vi "TCP Named Service - Server.vi"() -> ()   [LabVIEW 2015]
doc: "Creates a named service and listens on the first available port. When a client connects to the service, it sends a response string to the client."
panel:
  in  "MirrorCoverMotor":T1
  in  "Message to Send":string="You are currently accessing TCP Named Service - Server.vi from client %s on port %d."
  in  "Stop":bool
  # "Overview: Demonstrates the use of the TCP functions to initialize a named TCP service that can send data to a client VI.\nInstructions:\n1. Run the VI.\n2. Open TCP Named Service - Client.vi and follow the instructions on its front panel.\n3. Click Stop to stop the VI."
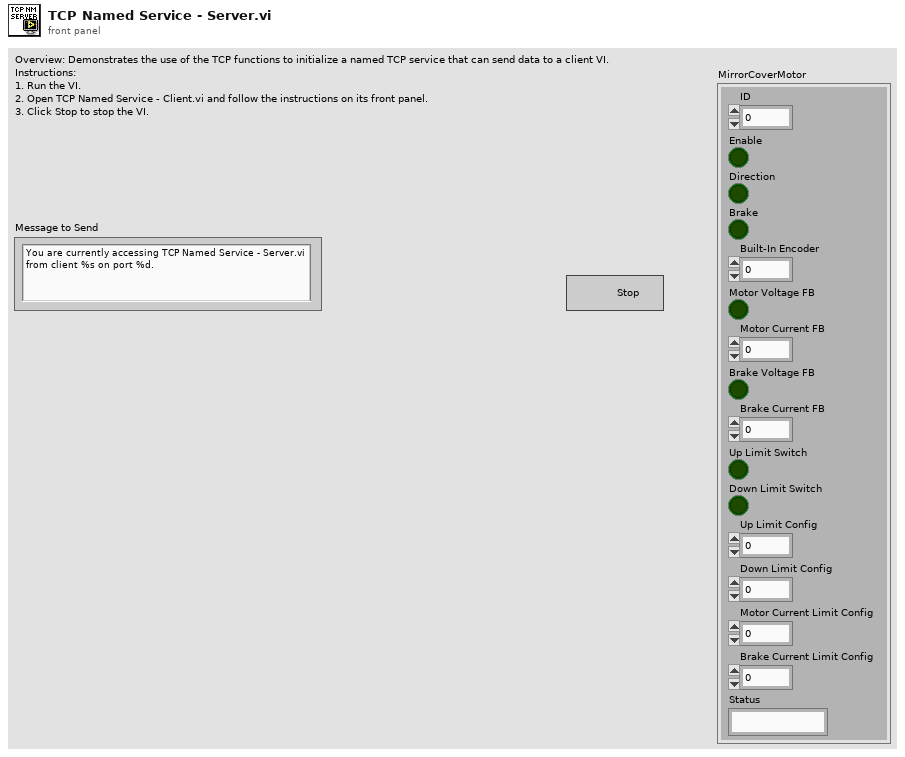
[diagram p1: front panel]
types:
  T1 = cluster{"ID":i32, "Enable":bool, "Direction":bool, "Brake":bool, "Built-In Encoder":u64, "Motor Voltage FB":bool, "Motor Current FB":u64, "Brake Voltage FB":bool, "Brake Current FB":u64, "Up Limit Switch":bool, "Down Limit Switch":bool, "Up Limit Config":u64, "Down Limit Config":u64, "Motor Current Limit Config":u64, "Brake Current Limit Config":u64, "Status":string}
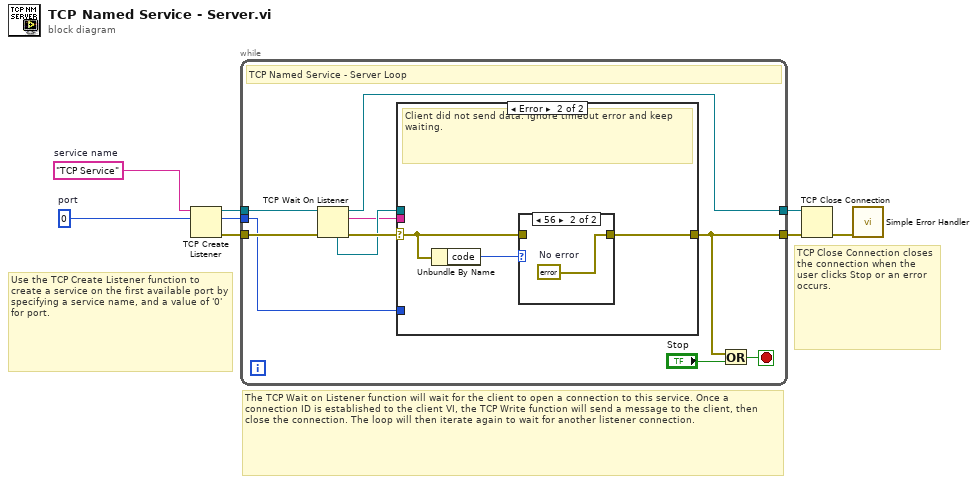
[diagram p0: block diagram]
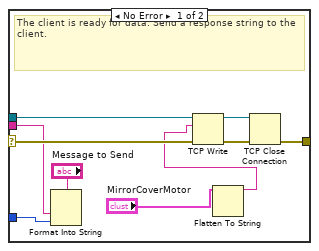
[diagram p2: hidden frame]
diagram:
  w2 = u16 0  # port
  w1 = "TCP Service"  # service name
  # "TCP Close Connection closes the connection when the user clicks Stop or an error occurs."
  # "The TCP Wait on Listener function will wait for the client to open a connection to this service. Once a connection ID is established to the client VI, the TCP Write function will send a message to the client, then close the connection. The loop will then iterate again to wait for another listener connection."
  # "Use the TCP Create Listener function to create a service on the first available port by specifying a service name, and a value of '0' for port."
  n1 = TCP Create Listener(10:w2, 11:w1) -> (0:w7:errorcluster, 2:w4:u16, 3:w8:refnum<k5>)  [unwired: 3 in]
  n2 = while {
    tunnel: [w11] -> w5
    tunnel: w8 -> [w18]
    tunnel: w7 -> [w16]
    tunnel: [w9] -> w6
    tunnel: w4 -> [w14]
    stop <- w13 stop-if-true
    # "TCP Named Service - Server Loop"
    n3 = TCP Wait On Listener(8:w16, 11:w18) -> (0:w17:errorcluster, 2:w10:string, 3:w9:refnum<k5>, 4:w15:refnum<k5>)  [unwired: 2 in, 1 out]
    n4 = case shown="Error" w17 {
      selector: w17 -> [w28 w31]
      tunnel: [w23 w29] -> w11
      tunnel: w15 -> [w26 _]
      tunnel: w14 -> [w27 _]
      tunnel: w10 -> [w25 _]
      frame No Error {
        # "The client is ready for data. Send a response string to the client."
        n5 = Format Into String(initial string="Message to Send", w25, w27) -> ()  [unwired: 2 in, 2 out]
        n6 = Flatten To String(anything="MirrorCoverMotor") -> (data string=w19:string)  [unwired: 3 in, 2 out]
        n7 = TCP Write(connection ID=w26, data in=w19, error in (no error)=w28) -> (connection ID out=w22:refnum<k5>, error out=w24:errorcluster)  [unwired: 1 in, 1 out]
        n8 = TCP Close Connection(connection ID=w22, error in (no error)=w24) -> (error out=w23:errorcluster)  [unwired: 1 in, 1 out]
      }
      frame Error {
        # "Client did not send data. Ignore timeout error and keep waiting."
        n9 = Unbundle By Name(w31) -> ("code"=w30:i32)
        n10 = case shown="56" w30 {
          tunnel: w31 -> [w32 _]
          tunnel: [w32 w33] -> w29
          frame Default {
          }
          frame 56 {
            w33 = errorcluster {"status"=FALSE, "code"=0, "source"=""}  # No error
          }
        }
      }
    }
    n11 = Or(x=w11, y="Stop") -> (x .or. y?=w13:bool)
  }
  n12 = TCP Close Connection(connection ID=w6, error in (no error)=w5) -> (error out=w3:errorcluster)  [unwired: 1 in, 1 out]
  n13 = call <vilib>:"Simple Error Handler.vi"("error in (no error)"=w3) -> ()  [unwired: 4 in, 5 out]
